vi "BottomStacking.vi"() -> ()   [LabVIEW 2014]
uses:
  BottomStacking.ctl
panel:
  in  "Activating Button":bool
  in  "State Machine":T1
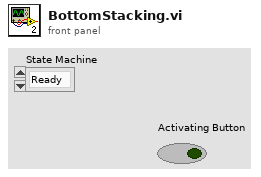
[diagram p1: front panel]
types:
  T1 = typedef "BottomStacking.ctl" = enum16{"Ready", "Raise To Stack Height", "Eject Internal Stack", "Set Down On Stack", "Release Tote", "Back Away", "Reset"}
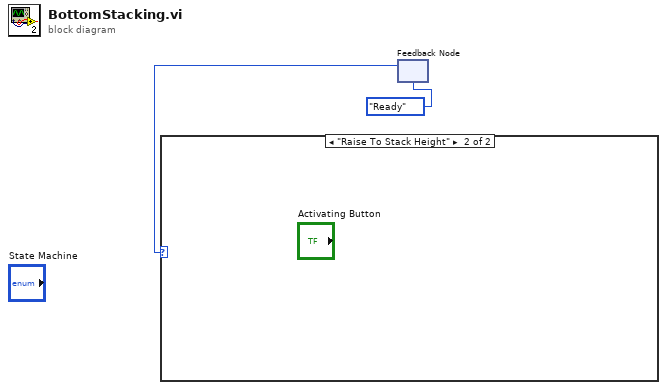
[diagram p0: block diagram]
diagram:
  n1 = feedback-in #1() -> ()  [unwired: 1 out]
  n2 = feedback #1(BottomStacking."Ready" ("State Machine")) -> (w1:T1)
  n3 = case shown="\"Raise To Stack Height\"" w1 {
    frame "Ready", Default {
    }
    frame "Raise To Stack Height" {
    }
  }
